vi "cm_Reset Peak Value.vi"(4 "Reset Peak?":bool, 7 "Display State In":T1={"Chan"=[], "First Drop?"=FALSE, "Notifier Name"="", "Refresh View"=FALSE, "Scale to Input Range"=FALSE, "Linear View"=FALSE, "Display"={"Current"=6618880, "Peak"=6618880}, "Property/Method"=enum."No Update", "Time Display Ref"=[]}) -> (2 "Display State Out":T1={"Chan"=[], "First Drop?"=FALSE, "Notifier Name"="", "Refresh View"=FALSE, "Scale to Input Range"=FALSE, "Linear View"=FALSE, "Display"={"Current"=6618880, "Peak"=6618880}, "Property/Method"=enum."No Update", "Time Display Ref"=[]})   [LabVIEW 2012, in "Channel Monitor.xctl"]
uses:
  Channel Monitor.xctl
  cm_Channel Monitor State.ctl
  TypeDef/cm_Property_Method.ctl
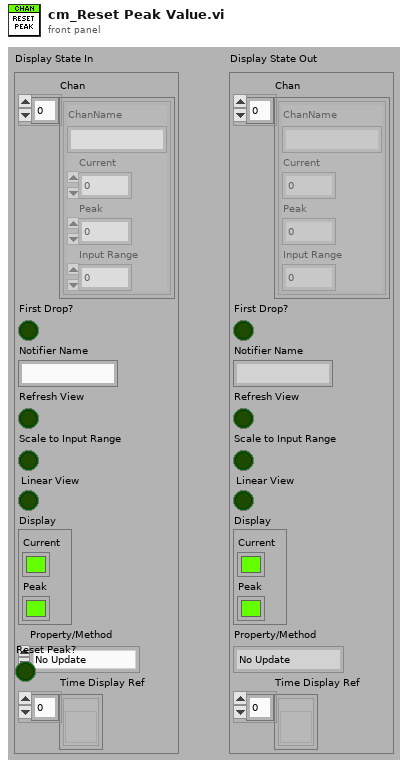
[diagram p1: front panel]
types:
  T1 = typedef "Channel Monitor.xctl/cm_Channel Monitor State.ctl" = cluster{"Chan":cluster{"ChanName":string, "Current":dbl, "Peak":dbl, "Input Range":dbl}[], "First Drop?":bool, "Notifier Name":string, "Refresh View":bool, "Scale to Input Range":bool, "Linear View":bool, "Display":cluster{"Current":u32, "Peak":u32}, "Property/Method":T2, "Time Display Ref":refnum<vi>[]}
  T2 = typedef "Channel Monitor.xctl/cm_Property_Method.ctl" = enum16{"No Update", "Color: Currrent", "Color: Peak", "Close Time Displays"}
  T3 = cluster{"ChanName":string, "Current":dbl, "Peak":dbl, "Input Range":dbl}[]
  T4 = cluster{"ChanName":string, "Current":dbl, "Peak":dbl, "Input Range":dbl}
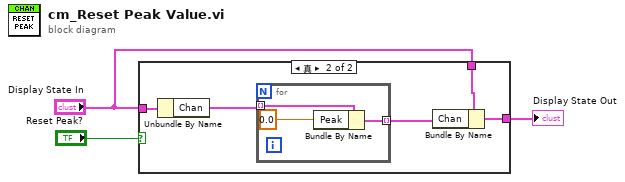
[diagram p0: block diagram]
diagram:
  n1 = case shown="真" "Reset Peak?" {
    tunnel: [w4 w9] -> w3
    tunnel: "Display State In" -> [w4 w7]
    tunnel: "Display State In" -> [_ w5]
    frame False {
    }
    frame True {
      n2 = Unbundle By Name(w5) -> ("Chan"=w6:T3)
      n3 = for {
        tunnel: w6 -> [w12] mode=indexing
        tunnel: [w11] -> w8 mode=indexing
        n4 = Bundle By Name(cluster=w12, "Peak"=0.0) -> (w11:T4)
      }
      n5 = Bundle By Name(cluster=w7, "Chan"=w8) -> (w9:T1)
    }
  }
  "Display State Out" <- w3
